vi "Read Results from processing.vi"(8 "error in":errorcluster, 11 "WaveformAcq runtime in":refnum<class "WaveformAcq runtime.lvclass">) -> (0 "error out":errorcluster, 2 "Results from processing":T1, 3 "WaveformAcq runtime out":refnum<class "WaveformAcq runtime.lvclass">)   [LabVIEW 2017, in "WaveformAcq runtime.lvclass"]
uses:
  WaveformAcq runtime.lvclass
  configuration/result data indices.ctl
  WaveformAcq runtime.lvclass/WaveformAcq runtime.ctl
  configuration/WaveformAcq configuration.lvclass
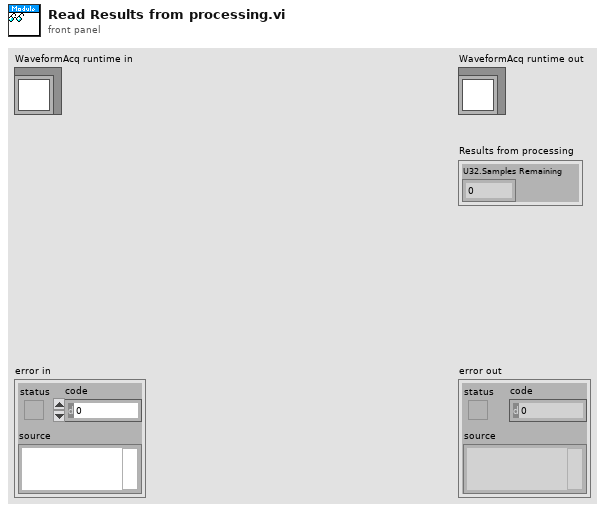
[diagram p1: front panel]
types:
  T1 = typedef "WaveformAcq configuration.lvclass/result data indices.ctl" = cluster{"U32.Samples Remaining":i32}
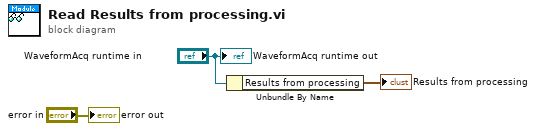
[diagram p0: block diagram]
diagram:
  n1 = Unbundle By Name("WaveformAcq runtime in") -> ("Results from processing"=→"Results from processing":T1)
  "error out" <- "error in"
  "WaveformAcq runtime out" <- "WaveformAcq runtime in"
